vi "toml_list_sections.vi"(4 "vi":refnum<vi>, 8 "error in (no error)":errorcluster, 11 "path in":path) -> (0 "error out":errorcluster, 1 "sections":string[](array[string]), 2 "file loaded":bool, 3 "path out":path)   [LabVIEW 2017]
uses:
  <vilib>/Utility/error.llb/Clear Errors.vi
  toml_lock_obtain.vi
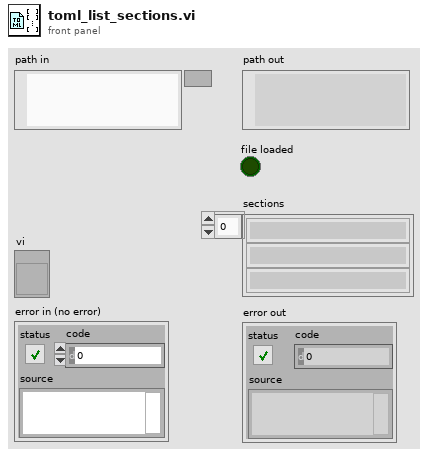
[diagram p1: front panel]
types:
  T1 = enum16{"open", "replace", "create", "open or create", "replace or create", "replace or create with confirmation"}
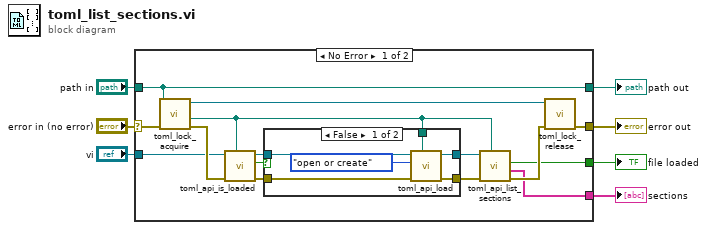
[diagram p0: block diagram]
diagram:
  n1 = case shown="No Error" "error in (no error)" {
    selector: "error in (no error)" -> [w21 w31]
    tunnel: [w20 w31] -> w6
    tunnel: "vi" -> [w17 _]
    tunnel: "path in" -> [w19 w32]
    tunnel: [w19 w32] -> w3
    tunnel: [w10 _] -> w2
    tunnel: [w9 _] -> w1
    frame No Error {
      n2 = call "toml_lock_acquire.vi"("error in (no error)"=w21, "path in"=w19) -> ("error out"=w18:errorcluster, "resolved path"=w8:path, "lock"=w22:refnum<queue>)  [unwired: 7 in]
      n3 = call "toml_api_is_loaded.vi"("resolved path"=w8, "error in (no error)"=w18, "vi in"=w17) -> ("error out"=w15:errorcluster, "file loaded"=w16:bool, "vi out"=w14:refnum<vi>)  [unwired: 5 in, 1 out]
      n4 = case shown="False" w16 {
        tunnel: w15 -> [w28 w30]
        tunnel: [w27 w30] -> w13
        tunnel: w8 -> [w24 _]
        tunnel: w14 -> [w26 w29]
        tunnel: [w25 w29] -> w12
        frame False {
          n5 = call "toml_api_load.vi"("resolved path"=w24, "error in (no error)"=w28, "operation"=T1."open or create" ("operation (open or create)"), "vi in"=w26) -> ("error out"=w27:errorcluster, "vi out"=w25:refnum<vi>)  [unwired: 5 in, 1 out]
        }
        frame True {
        }
      }
      n6 = call "toml_api_list_sections.vi"("resolved path"=w8, "error in (no error)"=w13, "vi in"=w12) -> ("error out"=w11:errorcluster, "sections"=w9:string[], "file loaded"=w10:bool)  [unwired: 5 in, 1 out]
      n7 = call "toml_lock_release.vi"("error in (no error)"=w11, "lock"=w22) -> ("error out"=w20:errorcluster)  [unwired: 9 in]
    }
    frame Error {
    }
  }
  "error out" <- w6
  "path out" <- w3
  "file loaded" <- w2
  "sections" <- w1
